vi "Read ConvBox.vi"(8 "error in":errorcluster, 9 "byte count":i32, 10 "address string":string, 11 "VISA resource in":refnum<visa-resource-name>) -> (0 "error out":errorcluster, 1 "ibsta":T1, 2 "data":string, 3 "VISA resource out":refnum<visa-resource-name>)   [LabVIEW 2023, in "Protocols.lvlib" / "RS-xxx to GPIB ConvBox.lvclass"]
uses:
  RS-xxx to GPIB ConvBox.lvclass
  <vilib>/Instr/_visa.llb/GPIB Status Boolean Array.ctl
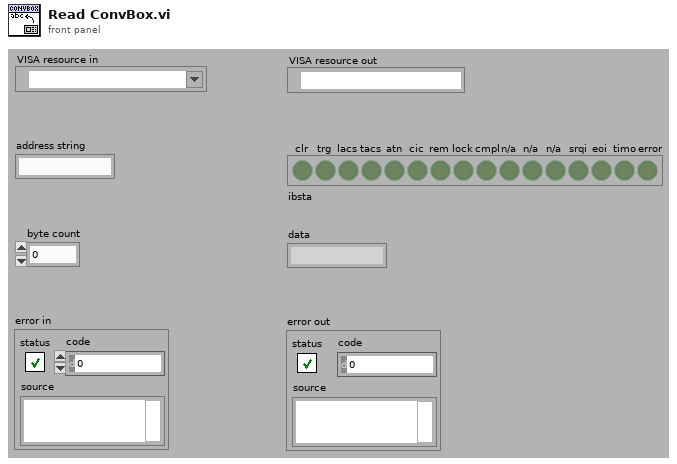
[diagram p1: front panel]
types:
  T1 = typedef "GPIB Status Boolean Array.ctl" = bool[]
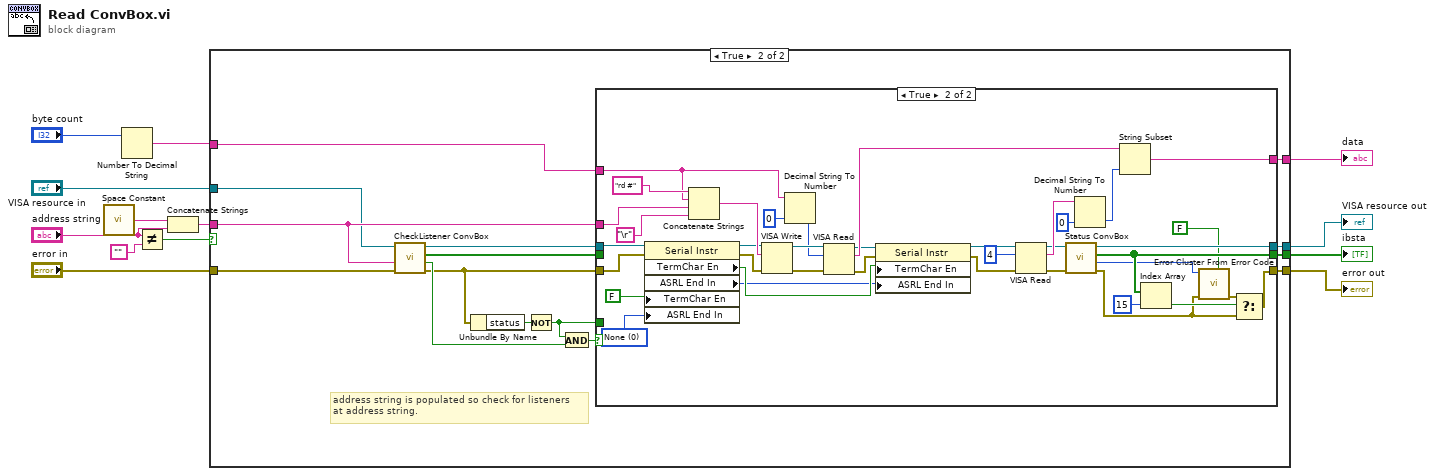
[diagram p0: block diagram]
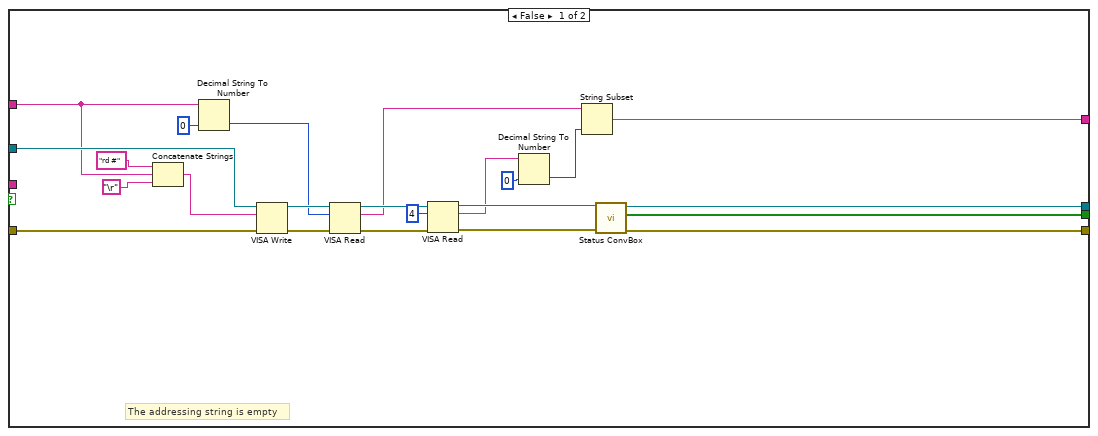
[diagram p2: hidden frame]
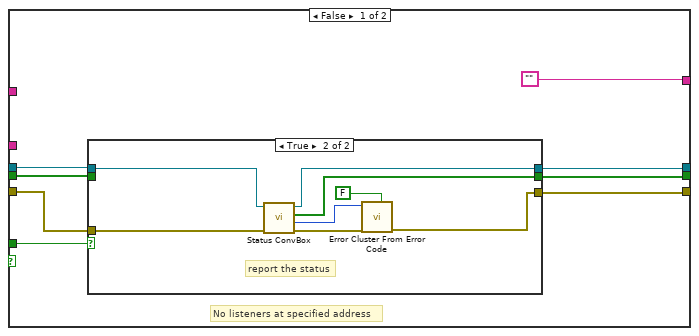
[diagram p3: hidden frame]
diagram:
  n1 = call <vilib>:"Space Constant.vi"() -> ("String"=w13:string)
  n2 = Number To Decimal String(number="byte count") -> (decimal integer string=w8:string)  [unwired: 1 in]
  n3 = Not Equal?(x="address string", y="") -> (x != y?=w5:bool)
  n4 = Concatenate Strings(w13, "address string") -> (w6:string)
  n5 = case shown="True" w5 {
    tunnel: [w31 w51] -> w3
    tunnel: [w30 w50] -> w2
    tunnel: [w29 w49] -> w1
    tunnel: w6 -> [_ w46]
    tunnel: "error in" -> [w34 w48]
    tunnel: "VISA resource in" -> [w33 w45]
    tunnel: w8 -> [w22 w44]
    tunnel: [w14 w37] -> w4
    frame False {
      # "The addressing string is empty"
      n6 = Concatenate Strings("rd #", w22, "\r") -> (w32:string)
      n7 = Decimal String To Number(string=w22, default (0L)=u32 0 ("default (0 I32)")) -> (number=w21:u32)  [unwired: 1 in, 1 out]
      n8 = VISA Write(VISA resource name=w33, write buffer=w32, error in (no error)=w34) -> (VISA resource name out=w25:refnum<visa-resource-name>, error out=w27:errorcluster)  [unwired: 1 out]
      n9 = VISA Read(VISA resource name=w25, byte count=w21, error in (no error)=w27) -> (VISA resource name out=w24:refnum<visa-resource-name>, read buffer=w15:string, error out=w28:errorcluster)  [unwired: 1 out]
      n10 = VISA Read(VISA resource name=w24, byte count=u32 4, error in (no error)=w28) -> (VISA resource name out=w23:refnum<visa-resource-name>, read buffer=w16:string, error out=w26:errorcluster)  [unwired: 1 out]
      n11 = Decimal String To Number(string=w16, default (0L)=u32 0 ("default (0 I32)")) -> (number=w17:u32)  [unwired: 1 in, 1 out]
      n12 = String Subset(string=w15, length (rest)=w17) -> (substring=w14:string)  [unwired: 1 in]
      n13 = call "Status ConvBox.vi"("error in (no error)"=w26, "VISA resource name"=w23) -> ("error out"=w29:errorcluster, "ibsta"=w30:T1, "VISA resource out"=w31:refnum<visa-resource-name>)  [unwired: 6 in, 1 out]
    }
    frame True {
      # "address string is populated so check for listeners\nat address string."
      n14 = call "CheckListener ConvBox.vi"("error in"=w48, "address string"=w46, "VISA resource in"=w45) -> ("error out"=w41:errorcluster, "listener found"=w42:bool, "ibsta"=w38:T1, "VISA resource out"=w47:refnum<visa-resource-name>)  [unwired: 5 in]
      n15 = Unbundle By Name(w41) -> ("status"=w43:bool)
      n16 = Not(x=w43) -> (.not. x?=w39:bool)
      n17 = And(x=w39, y=w42) -> (x .and. y?=w40:bool)
      n18 = case shown="True" w40 {
        tunnel: [w54 w108] -> w51
        tunnel: [w55 w93] -> w50
        tunnel: [w53 w87] -> w49
        tunnel: w41 -> [w57 w84]
        tunnel: w47 -> [w59 w83]
        tunnel: w46 -> [_ w98]
        tunnel: w44 -> [_ w101]
        tunnel: w39 -> [w58 _]
        tunnel: w38 -> [w56 _]
        tunnel: ["" w94] -> w37
        frame False {
          # "No listeners at specified address"
          n19 = case shown="True" w58 {
            tunnel: [w60 w69] -> w53
            tunnel: w57 -> [w60 w63]
            tunnel: w59 -> [w61 w64]
            tunnel: [w61 w67] -> w54
            tunnel: [w62 w65] -> w55
            tunnel: w56 -> [w62 _]
            frame False {
              # "Error reported by checklisteners"
            }
            frame True {
              # "report the status"
              n20 = call "Status ConvBox.vi"("error in (no error)"=w63, "VISA resource name"=w64) -> ("error out"=w68:errorcluster, "GPIB error"=w66:i16, "ibsta"=w65:T1, "VISA resource out"=w67:refnum<visa-resource-name>)  [unwired: 6 in]
              n21 = call <vilib>:"Error Cluster From Error Code.vi"("is warning? (False)"=FALSE, "error in (no error)"=w68, "error code (0)"=w66) -> ("error out"=w69:errorcluster)  [unwired: 6 in]
            }
          }
        }
        frame True {
          w77 = u16 0 items=["None", "Last Bit", "TermChar", "Break"] ("Serial Settings:End Mode for Writes")
          n22 = property class="Serial Instr"(reference=w83, error in=w84, "TermChar En"=FALSE ("Message Based Settings:Termination Character Enable"), "ASRL End In"=w77) -> (reference out=w82:refnum<visa-resource-name>, error out=w81:errorcluster, "TermChar En"=w80:bool, "ASRL End In"=w79:u16)
          n23 = Concatenate Strings("rd #", w101, w98, "\r") -> (w106:string)
          n24 = VISA Write(VISA resource name=w82, write buffer=w106, error in (no error)=w81) -> (VISA resource name out=w104:refnum<visa-resource-name>, error out=w103:errorcluster)  [unwired: 1 out]
          n25 = Decimal String To Number(string=w101, default (0L)=u32 0 ("default (0 I32)")) -> (number=w100:u32)  [unwired: 1 in, 1 out]
          n26 = VISA Read(VISA resource name=w104, byte count=w100, error in (no error)=w103) -> (VISA resource name out=w74:refnum<visa-resource-name>, read buffer=w85:string, error out=w73:errorcluster)  [unwired: 1 out]
          n27 = property class="Serial Instr"(reference=w74, error in=w73, "TermChar En"=w80, "ASRL End In"=w79) -> (reference out=w71:refnum<visa-resource-name>, error out=w72:errorcluster)
          n28 = VISA Read(VISA resource name=w71, byte count=u32 4 ("y"), error in (no error)=w72) -> (VISA resource name out=w76:refnum<visa-resource-name>, read buffer=w96:string, error out=w75:errorcluster)  [unwired: 1 out]
          n29 = call "Status ConvBox.vi"("error in (no error)"=w75, "VISA resource name"=w76) -> ("error out"=w90:errorcluster, "GPIB error"=w89:i16, "ibsta"=w93:T1, "VISA resource out"=w108:refnum<visa-resource-name>)  [unwired: 6 in]
          n30 = Decimal String To Number(string=w96, default (0L)=u32 0 ("default (0 I32)")) -> (number=w95:u32)  [unwired: 1 in, 1 out]
          n31 = String Subset(string=w85, length (rest)=w95) -> (substring=w94:string)  [unwired: 1 in]
          n32 = Index Array(array=w93, index=15) -> (element=w91:bool)
          n33 = call <vilib>:"Error Cluster From Error Code.vi"("is warning? (False)"=FALSE, "error in (no error)"=w90, "error code (0)"=w89) -> ("error out"=w88:errorcluster)  [unwired: 6 in]
          n34 = Select(t=w88, s=w91, f=w90) -> (s? t:f=w87:errorcluster)
        }
      }
    }
  }
  "data" <- w4
  "VISA resource out" <- w3
  "ibsta" <- w2
  "error out" <- w1
